vi "rsidr_core_global.vi"() -> ()   [LabVIEW 2020, in "Rohde&Schwarz CMWXP NR FR1 Measurement.lvlib"] (continued)
exceeding the specified power limits.\nDefault unit:  % \n\n<OffPowerBefore>\n float\nDefault unit:  dBm \n\n<OnPowerRMS>\n float\nDefault unit:  dBm \n\n<OnPowerPeak>\n float\nDefault unit:  dBm \n\n<OffPowerAfter>\n float\nDefault unit:  dBm\n\nAvailable Repeated Capabilities:\ninstance: i0, i1, i2, i3, i4, i5, i6, i7, i8, i9, i10, i11, i12, i13, i14, i15, i16, i17, i18, i19, i20, i21, i22, i23, i24, i25, i26, i27, i28, i29, i30, i31, i32\r\n\nRemote-control command(s):\nREAD:NRSub:MEAS<i>:MEValuation:PDYNamics:CURRent?"}, {"Level"=4, "Class Only"=FALSE, "Identifier"="RSCMWXPNRFR1M_ATTR_READ_MULTI_EVAL_MEAS_POWER_DYNAMICS_AVERAGE_RESULTS", "Descriptive Name"="Read Multi Eval Meas Power Dynamics Average Results", "Data Type"=enum."RawString", "Command"="READ:NRS:MEAS{instance}:MEV:PDYN:AVER?", "Access"=enum."Read Only", "Range Table"="", "Read Callback"="", "Write Callback"="", "Range Callback"="", "Check Callback"="", "Rngtable Callback"="", "Coerce Callback"="", "Supported Models"="", "Instrument Options"="", "Check Status Callback"="", "Flags"=0, "Help"="Return the average single value results of the power dynamics measurement.\n\nReturn values:  \n<Reliability>\n decimal\n\n<OutOfTolerance>\n decimal\nOut of tolerance result, i.e. percentage of measurement intervals of the statistic count for power dynamics measurements exceeding the specified power limits.\nDefault unit:  % \n\n<OffPowerBefore>\n float\nDefault unit:  dBm \n\n<OnPowerRMS>\n float\nDefault unit:  dBm \n\n<OnPowerPeak>\n float\nDefault unit:  dBm \n\n<OffPowerAfter>\n float\nDefault unit:  dBm\n\nAvailable Repeated Capabilities:\ninstance: i0, i1, i2, i3, i4, i5, i6, i7, i8, i9, i10, i11, i12, i13, i14, i15, i16, i17, i18, i19, i20, i21, i22, i23, i24, i25, i26, i27, i28, i29, i30, i31, i32\r\n\nRemote-control command(s):\nREAD:NRSub:MEAS<i>:MEValuation:PDYNamics:AVERage?"}, {"Level"=4, "Class Only"=FALSE, "Identifier"="RSCMWXPNRFR1M_ATTR_READ_MULTI_EVAL_MEAS_POWER_DYNAMICS_STANDARD_DEVIATION_RESULTS", "Descriptive Name"="Read Multi Eval Meas Power Dynamics Standard Deviation Results", "Data Type"=enum."RawString", "Command"="READ:NRS:MEAS{instance}:MEV:PDYN:SDEV?", "Access"=enum."Read Only", "Range Table"="", "Read Callback"="", "Write Callback"="", "Range Callback"="", "Check Callback"="", "Rngtable Callback"="", "Coerce Callback"="", "Supported Models"="", "Instrument Options"="", "Check Status Callback"="", "Flags"=0, "Help"="Return the standard deviation single value results of the power dynamics measurement.\n\nReturn values:  \n<Reliability>\n decimal\n\n<OutOfTolerance>\n decimal\nOut of tolerance result, i.e. percentage of measurement intervals of the statistic count for power dynamics measurements exceeding the specified power limits.\nDefault unit:  % \n\n<OffPowerBefore>\n float\nDefault unit:  dBm \n\n<OnPowerRMS>\n float\nDefault unit:  dBm \n\n<OnPowerPeak>\n float\nDefault unit:  dBm \n\n<OffPowerAfter>\n float\nDefault unit:  dBm\n\nAvailable Repeated Capabilities:\ninstance: i0, i1, i2, i3, i4, i5, i6, i7, i8, i9, i10, i11, i12, i13, i14, i15, i16, i17, i18, i19, i20, i21, i22, i23, i24, i25, i26, i27, i28, i29, i30, i31, i32\r\n\nRemote-control command(s):\nREAD:NRSub:MEAS<i>:MEValuation:PDYNamics:SDEViation?"}, {"Level"=4, "Class Only"=FALSE, "Identifier"="RSCMWXPNRFR1M_ATTR_READ_MULTI_EVAL_MEAS_POWER_DYNAMICS_MAXIMUM_RESULTS", "Descriptive Name"="Read Multi Eval Meas Power Dynamics Maximum Results", "Data Type"=enum."RawString", "Command"="READ:NRS:MEAS{instance}:MEV:PDYN:MAX?", "Access"=enum."Read Only", "Range Table"="", "Read Callback"="", "Write Callback"="", "Range Callback"="", "Check Callback"="", "Rngtable Callback"="", "Coerce Callback"="", "Supported Models"="", "Instrument Options"="", "Check Status Callback"="", "Flags"=0, "Help"="Return the maximum single value results of the power dynamics measurement.\n\nReturn values:  \n<Reliability>\n decimal\n\n<OutOfTolerance>\n decimal\nOut of tolerance result, i.e. percentage of measurement intervals of the statistic count for power dynamics measurements exceeding the specified power limits.\nDefault unit:  % \n\n<OffPowerBefore>\n float\nDefault unit:  dBm \n\n<OnPowerRMS>\n float\nDefault unit:  dBm \n\n<OnPowerPeak>\n float\nDefault unit:  dBm \n\n<OffPowerAfter>\n float\nDefault unit:  dBm\n\nAvailable Repeated Capabilities:\ninstance: i0, i1, i2, i3, i4, i5, i6, i7, i8, i9, i10, i11, i12, i13, i14, i15, i16, i17, i18, i19, i20, i21, i22, i23, i24, i25, i26, i27, i28, i29, i30, i31, i32\r\n\nRemote-control command(s):\nREAD:NRSub:MEAS<i>:MEValuation:PDYNamics:MAXimum?"}, {"Level"=4, "Class Only"=FALSE, "Identifier"="RSCMWXPNRFR1M_ATTR_READ_MULTI_EVAL_MEAS_POWER_DYNAMICS_MINIMUM_RESULTS", "Descriptive Name"="Read Multi Eval Meas Power Dynamics Minimum Results", "Data Type"=enum."RawString", "Command"="READ:NRS:MEAS{instance}:MEV:PDYN:MIN?", "Access"=enum."Read Only", "Range Table"="", "Read Callback"="", "Write Callback"="", "Range Callback"="", "Check Callback"="", "Rngtable Callback"="", "Coerce Callback"="", "Supported Models"="", "Instrument Options"="", "Check Status Callback"="", "Flags"=0, "Help"="Return the minimum single value results of the power dynamics measurement.\n\nReturn values:  \n<Reliability>\n decimal\n\n<OutOfTolerance>\n decimal\nOut of tolerance result, i.e. percentage of measurement intervals of the statistic count for power dynamics measurements exceeding the specified power limits.\nDefault unit:  % \n\n<OffPowerBefore>\n float\nDefault unit:  dBm \n\n<OnPowerRMS>\n float\nDefault unit:  dBm \n\n<OnPowerPeak>\n float\nDefault unit:  dBm \n\n<OffPowerAfter>\n float\nDefault unit:  dBm\n\nAvailable Repeated Capabilities:\ninstance: i0, i1, i2, i3, i4, i5, i6, i7, i8, i9, i10, i11, i12, i13, i14, i15, i16, i17, i18, i19, i20, i21, i22, i23, i24, i25, i26, i27, i28, i29, i30, i31, i32\r\n\nRemote-control command(s):\nREAD:NRSub:MEAS<i>:MEValuation:PDYNamics:MINimum?"}, {"Level"=4, "Class Only"=FALSE, "Identifier"="RSCMWXPNRFR1M_ATTR_FETCH_MULTI_EVAL_MEAS_POWER_DYNAMICS_CURRENT_RESULTS", "Descriptive Name"="Fetch Multi Eval Meas Power Dynamics Current Results", "Data Type"=enum."RawString", "Command"="FETC:NRS:MEAS{instance}:MEV:PDYN:CURR?", "Access"=enum."Read Only", "Range Table"="", "Read Callback"="", "Write Callback"="", "Range Callback"="", "Check Callback"="", "Rngtable Callback"="", "Coerce Callback"="", "Supported Models"="", "Instrument Options"="", "Check Status Callback"="", "Flags"=0, "Help"="Return the current single value results of the power dynamics measurement.\n\nReturn values:  \n<Reliability>\n decimal\n\n<OutOfTolerance>\n decimal\nOut of tolerance result, i.e. percentage of measurement intervals of the statistic count for power dynamics measurements exceeding the specified power limits.\nDefault unit:  % \n\n<OffPowerBefore>\n float\nDefault unit:  dBm \n\n<OnPowerRMS>\n float\nDefault unit:  dBm \n\n<OnPowerPeak>\n float\nDefault unit:  dBm \n\n<OffPowerAfter>\n float\nDefault unit:  dBm\n\nAvailable Repeated Capabilities:\ninstance: i0, i1, i2, i3, i4, i5, i6, i7, i8, i9, i10, i11, i12, i13, i14, i15, i16, i17, i18, i19, i20, i21, i22, i23, i24, i25, i26, i27, i28, i29, i30, i31, i32\r\n\nRemote-control command(s):\nFETCh:NRSub:MEAS<i>:MEValuation:PDYNamics:CURRent?"}, {"Level"=4, "Class Only"=FALSE, "Identifier"="RSCMWXPNRFR1M_ATTR_FETCH_MULTI_EVAL_MEAS_POWER_DYNAMICS_AVERAGE_RESULTS", "Descriptive Name"="Fetch Multi Eval Meas Power Dynamics Average Results", "Data Type"=enum."RawString", "Command"="FETC:NRS:MEAS{instance}:MEV:PDYN:AVER?", "Access"=enum."Read Only", "Range Table"="", "Read Callback"="", "Write Callback"="", "Range Callback"="", "Check Callback"="", "Rngtable Callback"="", "Coerce Callback"="", "Supported Models"="", "Instrument Options"="", "Check Status Callback"="", "Flags"=0, "Help"="Return the average single value results of the power dynamics measurement.\n\nReturn values:  \n<Reliability>\n decimal\n\n<OutOfTolerance>\n decimal\nOut of tolerance result, i.e. percentage of measurement intervals of the statistic count for power dynamics measurements exceeding the specified power limits.\nDefault unit:  % \n\n<OffPowerBefore>\n float\nDefault unit:  dBm \n\n<OnPowerRMS>\n float\nDefault unit:  dBm \n\n<OnPowerPeak>\n float\nDefault unit:  dBm \n\n<OffPowerAfter>\n float\nDefault unit:  dBm\n\nAvailable Repeated Capabilities:\ninstance: i0, i1, i2, i3, i4, i5, i6, i7, i8, i9, i10, i11, i12, i13, i14, i15, i16, i17, i18, i19, i20, i21, i22, i23, i24, i25, i26, i27, i28, i29, i30, i31, i32\r\n\nRemote-control command(s):\nFETCh:NRSub:MEAS<i>:MEValuation:PDYNamics:AVERage?"}, {"Level"=4, "Class Only"=FALSE, "Identifier"="RSCMWXPNRFR1M_ATTR_FETCH_MULTI_EVAL_MEAS_POWER_DYNAMICS_STANDARD_DEVIATION_RESULTS", "Descriptive Name"="Fetch Multi Eval Meas Power Dynamics Standard Deviation Results", "Data Type"=enum."RawString", "Command"="FETC:NRS:MEAS{instance}:MEV:PDYN:SDEV?", "Access"=enum."Read Only", "Range Table"="", "Read Callback"="", "Write Callback"="", "Range Callback"="", "Check Callback"="", "Rngtable Callback"="", "Coerce Callback"="", "Supported Models"="", "Instrument Options"="", "Check Status Callback"="", "Flags"=0, "Help"="Return the standard deviation single value results of the power dynamics measurement.\n\nReturn values:  \n<Reliability>\n decimal\n\n<OutOfTolerance>\n decimal\nOut of tolerance result, i.e. percentage of measurement intervals of the statistic count for power dynamics measurements exceeding the specified power limits.\nDefault unit:  % \n\n<OffPowerBefore>\n float\nDefault unit:  dBm \n\n<OnPowerRMS>\n float\nDefault unit:  dBm \n\n<OnPowerPeak>\n float\nDefault unit:  dBm \n\n<OffPowerAfter>\n float\nDefault unit:  dBm\n\nAvailable Repeated Capabilities:\ninstance: i0, i1, i2, i3, i4, i5, i6, i7, i8, i9, i10, i11, i12, i13, i14, i15, i16, i17, i18, i19, i20, i21, i22, i23, i24, i25, i26, i27, i28, i29, i30, i31, i32\r\n\nRemote-control command(s):\nFETCh:NRSub:MEAS<i>:MEValuation:PDYNamics:SDEViation?"}, {"Level"=4, "Class Only"=FALSE, "Identifier"="RSCMWXPNRFR1M_ATTR_FETCH_MULTI_EVAL_MEAS_POWER_DYNAMICS_MAXIMUM_RESULTS", "Descriptive Name"="Fetch Multi Eval Meas Power Dynamics Maximum Results", "Data Type"=enum."RawString", "Command"="FETC:NRS:MEAS{instance}:MEV:PDYN:MAX?", "Access"=enum."Read Only", "Range Table"="", "Read Callback"="", "Write Callback"="", "Range Callback"="", "Check Callback"="", "Rngtable Callback"="", "Coerce Callback"="", "Supported Models"="", "Instrument Options"="", "Check Status Callback"="", "Flags"=0, "Help"="Return the maximum single value results of the power dynamics measurement.\n\nReturn values:  \n<Reliability>\n decimal\n\n<OutOfTolerance>\n decimal\nOut of tolerance result, i.e. percentage of measurement intervals of the statistic count for power dynamics measurements exceeding the specified power limits.\nDefault unit:  % \n\n<OffPowerBefore>\n float\nDefault unit:  dBm \n\n<OnPowerRMS>\n float\nDefault unit:  dBm \n\n<OnPowerPeak>\n float\nDefault unit:  dBm \n\n<OffPowerAfter>\n float\nDefault unit:  dBm\n\nAvailable Repeated Capabilities:\ninstance: i0, i1, i2, i3, i4, i5, i6, i7, i8, i9, i10, i11, i12, i13, i14, i15, i16, i17, i18, i19, i20, i21, i22, i23, i24, i25, i26, i27, i28, i29, i30, i31, i32\r\n\nRemote-control command(s):\nFETCh:NRSub:MEAS<i>:MEValuation:PDYNamics:MAXimum?"}, {"Level"=4, "Class Only"=FALSE, "Identifier"="RSCMWXPNRFR1M_ATTR_FETCH_MULTI_EVAL_MEAS_POWER_DYNAMICS_MINIMUM_RESULTS", "Descriptive Name"="Fetch Multi Eval Meas Power Dynamics Minimum Results", "Data Type"=enum."RawString", "Command"="FETC:NRS:MEAS{instance}:MEV:PDYN:MIN?", "Access"=enum."Read Only", "Range Table"="", "Read Callback"="", "Write Callback"="", "Range Callback"="", "Check Callback"="", "Rngtable Callback"="", "Coerce Callback"="", "Supported Models"="", "Instrument Options"="", "Check Status Callback"="", "Flags"=0, "Help"="Return the minimum single value results of the power dynamics measurement.\n\nReturn values:  \n<Reliability>\n decimal\n\n<OutOfTolerance>\n decimal\nOut of tolerance result, i.e. percentage of measurement intervals of the statistic count for power dynamics measurements exceeding the specified power limits.\nDefault unit:  % \n\n<OffPowerBefore>\n float\nDefault unit:  dBm \n\n<OnPowerRMS>\n float\nDefault unit:  dBm \n\n<OnPowerPeak>\n float\nDefault unit:  dBm \n\n<OffPowerAfter>\n float\nDefault unit:  dBm\n\nAvailable Repeated Capabilities:\ninstance: i0, i1, i2, i3, i4, i5, i6, i7, i8, i9, i10, i11, i12, i13, i14, i15, i16, i17, i18, i19, i20, i21, i22, i23, i24, i25, i26, i27, i28, i29, i30, i31, i32\r\n\nRemote-control command(s):\nFETCh:NRSub:MEAS<i>:MEValuation:PDYNamics:MINimum?"}, {"Level"=3, "Class Only"=TRUE, "Identifier"="", "Descriptive Name"="List", "Data Type"=enum."ViInt32", "Command"="", "Access"=enum."Read Only", "Range Table"="", "Read Callback"="", "Write Callback"="", "Range Callback"="", "Check Callback"="", "Rngtable Callback"="", "Coerce Callback"="", "Supported Models"="", "Instrument Options"="", "Check Status Callback"="", "Flags"=0, "Help"="The attributes in this class return a selected list mode result for all measured segments. The number of returned results depends on the number of measured segments."}, {"Level"=4, "Class Only"=TRUE, "Identifier"="", "Descriptive Name"="ACLR Spectrum", "Data Type"=enum."ViInt32", "Command"="", "Access"=enum."Read Only", "Range Table"="", "Read Callback"="", "Write Callback"="", "Range Callback"="", "Check Callback"="", "Rngtable Callback"="", "Coerce Callback"="", "Supported Models"="", "Instrument Options"="", "Check Status Callback"="", "Flags"=0, "Help"="The attributes in this class return ACLR spectrum results for all measured segments. The number of returned results depends on the number of measured segments."}, {"Level"=5, "Class Only"=FALSE, "Identifier"="RSCMWXPNRFR1M_ATTR_FETCH_MULTI_EVAL_MEAS_LIST_ACLR_DETECTED_ALLOCATION_RESULTS", "Descriptive Name"="Fetch Multi Eval Meas List ACLR Detected Allocation Results", "Data Type"=enum."RawString", "Command"="FETC:NRS:MEAS{instance}:MEV:LIST:ACLR:DALL?", "Access"=enum."Read Only", "Range Table"="", "Read Callback"="", "Write Callback"="", "Range Callback"="", "Check Callback"="", "Rngtable Callback"="", "Coerce Callback"="", "Supported Models"="", "Instrument Options"="", "Check Status Callback"="", "Flags"=0, "Help"="Return the detected allocation for all measured list mode segments. The result is determined from the last measured slot of the statistical length of a segment. The individual measurements provide identical detected allocation results when measuring the same slot. However different statistical lengths can be defined for the measurements so that the measured slots and returned results can differ.\n\nThe results are returned as pairs per segment: <Reliability>, {<NrResBlocks>, <OffsetResBlocks>}seg 1, {<NrResBlocks>, <OffsetResBlocks>}seg 2, ...\n\nReturn values:  \n<Reliability>\n decimal\n\n<NrResBlocks>\n decimal\nNumber of allocated resource blocks\n\n<OffsetResBlocks>\n decimal\nOffset of the first allocated resource block from the edge of the allocated UL transmission bandwidth\n\nAvailable Repeated Capabilities:\ninstance: i0, i1, i2, i3, i4, i5, i6, i7, i8, i9, i10, i11, i12, i13, i14, i15, i16, i17, i18, i19, i20, i21, i22, i23, i24, i25, i26, i27, i28, i29, i30, i31, i32\r\n\nRemote-control command(s):\nFETCh:NRSub:MEAS<i>:MEValuation:LIST:ACLR:DALLocation?"}, {"Level"=5, "Class Only"=FALSE, "Identifier"="RSCMWXPNRFR1M_ATTR_FETCH_MULTI_EVAL_MEAS_LIST_ACLR_NR_CURRENT_RESULTS", "Descriptive Name"="Fetch Multi Eval Meas List ACLR NR Current Results", "Data Type"=enum."RawString", "Command"="FETC:NRS:MEAS{instance}:MEV:LIST:ACLR:NR:CURR?", "Access"=enum."Read Only", "Range Table"="", "Read Callback"="", "Write Callback"="", "Range Callback"="", "Check Callback"="", "Rngtable Callback"="", "Coerce Callback"="", "Supported Models"="", "Instrument Options"="", "Check Status Callback"="", "Flags"=0, "Help"="Return the power in the allocated NR channel for all measured list mode segments.\n\nReturn values:  \n<Reliability>\n decimal\n\n<Power>\n float\nComma-separated list of values, one per measured segment\nDefault unit:  dBm\n\nAvailable Repeated Capabilities:\ninstance: i0, i1, i2, i3, i4, i5, i6, i7, i8, i9, i10, i11, i12, i13, i14, i15, i16, i17, i18, i19, i20, i21, i22, i23, i24, i25, i26, i27, i28, i29, i30, i31, i32\r\n\nRemote-control command(s):\nFETCh:NRSub:MEAS<i>:MEValuation:LIST:ACLR:NR:CURRent?"}, {"Level"=5, "Class Only"=FALSE, "Identifier"="RSCMWXPNRFR1M_ATTR_FETCH_MULTI_EVAL_MEAS_LIST_ACLR_NR_AVERAGE_RESULTS", "Descriptive Name"="Fetch Multi Eval Meas List ACLR NR Average Results", "Data Type"=enum."RawString", "Command"="FETC:NRS:MEAS{instance}:MEV:LIST:ACLR:NR:AVER?", "Access"=enum."Read Only", "Range Table"="", "Read Callback"="", "Write Callback"="", "Range Callback"="", "Check Callback"="", "Rngtable Callback"="", "Coerce Callback"="", "Supported Models"="", "Instrument Options"="", "Check Status Callback"="", "Flags"=0, "Help"="Return the average power in the allocated NR channel for all measured list mode segments.\n\nReturn values:  \n<Reliability>\n decimal\n\n<Power>\n float\nComma-separated list of values, one per measured segment\nDefault unit:  dBm\n\nAvailable Repeated Capabilities:\ninstance: i0, i1, i2, i3, i4, i5, i6, i7, i8, i9, i10, i11, i12, i13, i14, i15, i16, i17, i18, i19, i20, i21, i22, i23, i24, i25, i26, i27, i28, i29, i30, i31, i32\r\n\nRemote-control command(s):\nFETCh:NRSub:MEAS<i>:MEValuation:LIST:ACLR:NR:AVERage?"}, {"Level"=5, "Class Only"=FALSE, "Identifier"="RSCMWXPNRFR1M_ATTR_QUERY_MULTI_EVAL_MEAS_LIST_ACLR_NR_CURRENT_LIMIT_CHECK_RESULTS", "Descriptive Name"="Query Multi Eval Meas List ACLR NR Current Limit Check Results", "Data Type"=enum."RawString", "Command"="CALC:NRS:MEAS{instance}:MEV:LIST:ACLR:NR:CURR?", "Access"=enum."Read Only", "Range Table"="", "Read Callback"="", "Write Callback"="", "Range Callback"="", "Check Callback"="", "Rngtable Callback"="", "Coerce Callback"="", "Supported Models"="", "Instrument Options"="", "Check Status Callback"="", "Flags"=0, "Help"="Return the power limit check results in the allocated NR channel for all measured list mode segments.\n\nReturn values:  \n<Reliability>\n decimal\n\n<PowerLimCheck>\n limit check result\nComma-separated list of results, one per measured segment\n\nAvailable Repeated Capabilities:\ninstance: i0, i1, i2, i3, i4, i5, i6, i7, i8, i9, i10, i11, i12, i13, i14, i15, i16, i17, i18, i19, i20, i21, i22, i23, i24, i25, i26, i27, i28, i29, i30, i31, i32\r\n\nRemote-control command(s):\nCALCulate:NRSub:MEAS<i>:MEValuation:LIST:ACLR:NR:CURRent?"}, {"Level"=5, "Class Only"=FALSE, "Identifier"="RSCMWXPNRFR1M_ATTR_QUERY_MULTI_EVAL_MEAS_LIST_ACLR_NR_AVERAGE_LIMIT_CHECK_RESULTS", "Descriptive Name"="Query Multi Eval Meas List ACLR NR Average Limit Check Results", "Data Type"=enum."RawString", "Command"="CALC:NRS:MEAS{instance}:MEV:LIST:ACLR:NR:AVER?", "Access"=enum."Read Only", "Range Table"="", "Read Callback"="", "Write Callback"="", "Range Callback"="", "Check Callback"="", "Rngtable Callback"="", "Coerce Callback"="", "Supported Models"="", "Instrument Options"="", "Check Status Callback"="", "Flags"=0, "Help"="Return the average \tpower limit check results in the allocated NR channel for all measured list mode segments.\n\nReturn values:  \n<Reliability>\n decimal\n\n<PowerLimCheck>\n limit check result\nComma-separated list of results, one per measured segment\n\nAvailable Repeated Capabilities:\ninstance: i0, i1, i2, i3, i4, i5, i6, i7, i8, i9, i10, i11, i12, i13, i14, i15, i16, i17, i18, i19, i20, i21, i22, i23, i24, i25, i26, i27, i28, i29, i30, i31, i32\r\n\nRemote-control command(s):\nCALCulate:NRSub:MEAS<i>:MEValuation:LIST:ACLR:NR:AVERage?"}, {"Level"=5, "Class Only"=FALSE, "Identifier"="RSCMWXPNRFR1M_ATTR_FETCH_MULTI_EVAL_MEAS_LIST_ACLR_NR_NEGATIVE_CURRENT_RESULTS", "Descriptive Name"="Fetch Multi Eval Meas List ACLR NR Negative Current Results", "Data Type"=enum."RawString", "Command"="FETC:NRS:MEAS{instance}:MEV:LIST:ACLR:NR:NEG:CURR?", "Access"=enum."Read Only", "Range Table"="", "Read Callback"="", "Write Callback"="", "Range Callback"="", "Check Callback"="", "Rngtable Callback"="", "Coerce Callback"="", "Supported Models"="", "Instrument Options"="", "Check Status Callback"="", "Flags"=0, "Help"="Return the ACLR for the first adjacent NR channel below (Negative) the carrier frequency for all measured list mode segments.\n\nReturn values:  \n<Reliability>\n decimal\n\n<ACLR>\n float\nComma-separated list of values, one per measured segment\nDefault unit:  dB\n\nAvailable Repeated Capabilities:\ninstance: i0, i1, i2, i3, i4, i5, i6, i7, i8, i9, i10, i11, i12, i13, i14, i15, i16, i17, i18, i19, i20, i21, i22, i23, i24, i25, i26, i27, i28, i29, i30, i31, i32\r\n\nRemote-control command(s):\nFETCh:NRSub:MEAS<i>:MEValuation:LIST:ACLR:NR:NEGativ:CURRent?"}, {"Level"=5, "Class Only"=FALSE, "Identifier"="RSCMWXPNRFR1M_ATTR_FETCH_MULTI_EVAL_MEAS_LIST_ACLR_NR_NEGATIVE_AVERAGE_RESULTS", "Descriptive Name"="Fetch Multi Eval Meas List ACLR NR Negative Average Results", "Data Type"=enum."RawString", "Command"="FETC:NRS:MEAS{instance}:MEV:LIST:ACLR:NR:NEG:AVER?", "Access"=enum."Read Only", "Range Table"="", "Read Callback"="", "Write Callback"="", "Range Callback"="", "Check Callback"="", "Rngtable Callback"="", "Coerce Callback"="", "Supported Models"="", "Instrument Options"="", "Check Status Callback"="", "Flags"=0, "Help"="Return the average ACLR for the first adjacent NR channel below (Negative) the carrier frequency for all measured list mode segments.\n\nReturn values:  \n<Reliability>\n decimal\n\n<ACLR>\n float\nComma-separated list of values, one per measured segment\nDefault unit:  dB\n\nAvailable Repeated Capabilities:\ninstance: i0, i1, i2, i3, i4, i5, i6, i7, i8, i9, i10, i11, i12, i13, i14, i15, i16, i17, i18, i19, i20, i21, i22, i23, i24, i25, i26, i27, i28, i29, i30, i31, i32\r\n\nRemote-control command(s):\nFETCh:NRSub:MEAS<i>:MEValuation:LIST:ACLR:NR:NEGativ:AVERage?"}, {"Level"=5, "Class Only"=FALSE, "Identifier"="RSCMWXPNRFR1M_ATTR_FETCH_MULTI_EVAL_MEAS_LIST_ACLR_NR_POSITIVE_CURRENT_RESULTS", "Descriptive Name"="Fetch Multi Eval Meas List ACLR NR Positive Current Results", "Data Type"=enum."RawString", "Command"="FETC:NRS:MEAS{instance}:MEV:LIST:ACLR:NR:POS:CURR?", "Access"=enum."Read Only", "Range Table"="", "Read Callback"="", "Write Callback"="", "Range Callback"="", "Check Callback"="", "Rngtable Callback"="", "Coerce Callback"="", "Supported Models"="", "Instrument Options"="", "Check Status Callback"="", "Flags"=0, "Help"="Return the ACLR for the first adjacent NR channel above (Positive) the carrier frequency for all measured list mode segments.\n\nReturn values:  \n<Reliability>\n decimal\n\n<ACLR>\n float\nComma-separated list of values, one per measured segment\nDefault unit:  dB\n\nAvailable Repeated Capabilities:\ninstance: i0, i1, i2, i3, i4, i5, i6, i7, i8, i9, i10, i11, i12, i13, i14, i15, i16, i17, i18, i19, i20, i21, i22, i23, i24, i25, i26, i27, i28, i29, i30, i31, i32\r\n\nRemote-control command(s):\nFETCh:NRSub:MEAS<i>:MEValuation:LIST:ACLR:NR:POSitiv:CURRent?"}, {"Level"=5, "Class Only"=FALSE, "Identifier"="RSCMWXPNRFR1M_ATTR_FETCH_MULTI_EVAL_MEAS_LIST_ACLR_NR_POSITIVE_AVERAGE_RESULTS", "Descriptive Name"="Fetch Multi Eval Meas List ACLR NR Positive Average Results", "Data Type"=enum."RawString", "Command"="FETC:NRS:MEAS{instance}:MEV:LIST:ACLR:NR:POS:AVER?", "Access"=enum."Read Only", "Range Table"="", "Read Callback"="", "Write Callback"="", "Range Callback"="", "Check Callback"="", "Rngtable Callback"="", "Coerce Callback"="", "Supported Models"="", "Instrument Options"="", "Check Status Callback"="", "Flags"=0, "Help"="Return the average ACLR for the first adjacent NR channel above (Positive) the carrier frequency for all measured list mode segments.\n\nReturn values:  \n<Reliability>\n decimal\n\n<ACLR>\n float\nComma-separated list of values, one per measured segment\nDefault unit:  dB\n\nAvailable Repeated Capabilities:\ninstance: i0, i1, i2, i3, i4, i5, i6, i7, i8, i9, i10, i11, i12, i13, i14, i15, i16, i17, i18, i19, i20, i21, i22, i23, i24, i25, i26, i27, i28, i29, i30, i31, i32\r\n\nRemote-control command(s):\nFETCh:NRSub:MEAS<i>:MEValuation:LIST:ACLR:NR:POSitiv:AVERage?"}, {"Level"=5, "Class Only"=FALSE, "Identifier"="RSCMWXPNRFR1M_ATTR_QUERY_MULTI_EVAL_MEAS_LIST_ACLR_NR_NEGATIVE_CURRENT_LIMIT_CHECK_RESULTS", "Descriptive Name"="Query Multi Eval Meas List ACLR NR Negative Current Limit Check Results", "Data Type"=enum."RawString", "Command"="CALC:NRS:MEAS{instance}:MEV:LIST:ACLR:NR:NEG:CURR?", "Access"=enum."Read Only", "Range Table"="", "Read Callback"="", "Write Callback"="", "Range Callback"="", "Check Callback"="", "Rngtable Callback"="", "Coerce Callback"="", "Supported Models"="", "Instrument Options"="", "Check Status Callback"="", "Flags"=0, "Help"="Return the ACLR limit check results for the first adjacent NR channel below (Negative) the carrier frequency for all measured list mode segments.\n\nReturn values:  \n<Reliability>\n decimal\n\n<ACLRLimCheck>\n limit check result\nComma-separated list of values, one per measured segment\n\nAvailable Repeated Capabilities:\ninstance: i0, i1, i2, i3, i4, i5, i6, i7, i8, i9, i10, i11, i12, i13, i14, i15, i16, i17, i18, i19, i20, i21, i22, i23, i24, i25, i26, i27, i28, i29, i30, i31, i32\r\n\nRemote-control command(s):\nCALCulate:NRSub:MEAS<i>:MEValuation:LIST:ACLR:NR:NEGativ:CURRent?"}, {"Level"=5, "Class Only"=FALSE, "Identifier"="RSCMWXPNRFR1M_ATTR_QUERY_MULTI_EVAL_MEAS_LIST_ACLR_NR_NEGATIVE_AVERAGE_LIMIT_CHECK_RESULTS", "Descriptive Name"="Query Multi Eval Meas List ACLR NR Negative Average Limit Check Results", "Data Type"=enum."RawString", "Command"="CALC:NRS:MEAS{instance}:MEV:LIST:ACLR:NR:NEG:AVER?", "Access"=enum."Read Only", "Range Table"="", "Read Callback"="", "Write Callback"="", "Range Callback"="", "Check Callback"="", "Rngtable Callback"="", "Coerce Callback"="", "Supported Models"="", "Instrument Options"="", "Check Status Callback"="", "Flags"=0, "Help"="Return the average ACLR limit check results for the first adjacent NR channel below (Negative) the carrier frequency for all measured list mode segments.\n\nReturn values:  \n<Reliability>\n decimal\n\n<ACLRLimCheck>\n limit check result\nComma-separated list of values, one per measured segment\n\nAvailable Repeated Capabilities:\ninstance: i0, i1, i2, i3, i4, i5, i6, i7, i8, i9, i10, i11, i12, i13, i14, i15, i16, i17, i18, i19, i20, i21, i22, i23, i24, i25, i26, i27, i28, i29, i30, i31, i32\r\n\nRemote-control command(s):\nCALCulate:NRSub:MEAS<i>:MEValuation:LIST:ACLR:NR:NEGativ:AVERage?"}, {"Level"=5, "Class Only"=FALSE, "Identifier"="RSCMWXPNRFR1M_ATTR_QUERY_MULTI_EVAL_MEAS_LIST_ACLR_NR_POSITIVE_CURRENT_LIMIT_CHECK_RESULTS", "Descriptive Name"="Query Multi Eval Meas List ACLR NR Positive Current Limit Check Results", "Data Type"=enum."RawString", "Command"="CALC:NRS:MEAS{instance}:MEV:LIST:ACLR:NR:POS:CURR?", "Access"=enum."Read Only", "Range Table"="", "Read Callback"="", "Write Callback"="", "Range Callback"="", "Check Callback"="", "Rngtable Callback"="", "Coerce Callback"="", "Supported Models"="", "Instrument Options"="", "Check Status Callback"="", "Flags"=0, "Help"="Return the ACLR limit check results for the first adjacent NR channel above (Positive) the carrier frequency for all measured list mode segments.\n\nReturn values:  \n<Reliability>\n decimal\n\n<ACLRLimCheck>\n limit check result\nComma-separated list of values, one per measured segment\n\nAvailable Repeated Capabilities:\ninstance: i0, i1, i2, i3, i4, i5, i6, i7, i8, i9, i10, i11, i12, i13, i14, i15, i16, i17, i18, i19, i20, i21, i22, i23, i24, i25, i26, i27, i28, i29, i30, i31, i32\r\n\nRemote-control command(s):\nCALCulate:NRSub:MEAS<i>:MEValuation:LIST:ACLR:NR:POSitiv:CURRent?"}, {"Level"=5, "Class Only"=FALSE, "Identifier"="RSCMWXPNRFR1M_ATTR_QUERY_MULTI_EVAL_MEAS_LIST_ACLR_NR_POSITIVE_AVERAGE_LIMIT_CHECK_RESULTS", "Descriptive Name"="Query Multi Eval Meas List ACLR NR Positive Average Limit Check Results", "Data Type"=enum."RawString", "Command"="CALC:NRS:MEAS{instance}:MEV:LIST:ACLR:NR:POS:AVER?", "Access"=enum."Read Only", "Range Table"="", "Read Callback"="", "Write Callback"="", "Range Callback"="", "Check Callback"="", "Rngtable Callback"="", "Coerce Callback"="", "Supported Models"="", "Instrument Options"="", "Check Status Callback"="", "Flags"=0, "Help"="Return the average ACLR limit check results for the first adjacent NR channel above (Positive) the carrier frequency for all measured list mode segments.\n\nReturn values:  \n<Reliability>\n decimal\n\n<ACLRLimCheck>\n limit check result\nComma-separated list of values, one per measured segment\n\nAvailable Repeated Capabilities:\ninstance: i0, i1, i2, i3, i4, i5, i6, i7, i8, i9, i10, i11, i12, i13, i14, i15, i16, i17, i18, i19, i20, i21, i22, i23, i24, i25, i26, i27, i28, i29, i30, i31, i32\r\n\nRemote-control command(s):\nCALCulate:NRSub:MEAS<i>:MEValuation:LIST:ACLR:NR:POSitiv:AVERage?"}, {"Level"=5, "Class Only"=TRUE, "Identifier"="", "Descriptive Name"="UTRA", "Data Type"=enum."ViInt32", "Command"="", "Access"=enum."Read Only", "Range Table"="", "Read Callback"="", "Write Callback"="", "Range Callback"="", "Check Callback"="", "Rngtable Callback"="", "Coerce Callback"="", "Supported Models"="", "Instrument Options"="", "Check Status Callback"="", "Flags"=0, "Help"="The attributes in this class return results for adjacent UTRA channels."}, {"Level"=6, "Class Only"=FALSE, "Identifier"="RSCMWXPNRFR1M_ATTR_FETCH_MULTI_EVAL_MEAS_LIST_ACLR_UTRA_NEGATIVE_CURRENT_RESULTS", "Descriptive Name"="Fetch Multi Eval Meas List ACLR UTRA Negative Current Results", "Data Type"=enum."RawString", "Command"="FETC:NRS:MEAS{instance}:MEV:LIST:ACLR:UTRA{UTRA}:NEG:CURR?", "Access"=enum."Read Only", "Range Table"="", "Read Callback"="", "Write Callback"="", "Range Callback"="", "Check Callback"="", "Rngtable Callback"="", "Coerce Callback"="", "Supported Models"="", "Instrument Options"="", "Check Status Callback"="", "Flags"=0, "Help"="Return the ACLR for the first or second adjacent UTRA channel below (Negative) the carrier frequency for all measured list mode segments.\n\nReturn values:  \n<Reliability>\n decimal\n\n<ACLR>\n float\nComma-separated list of values, one per measured segment\nDefault unit:  dB\n\nAvailable Repeated Capabilities:\ninstance: i0, i1, i2, i3, i4, i5, i6, i7, i8, i9, i10, i11, i12, i13, i14, i15, i16, i17, i18, i19, i20, i21, i22, i23, i24, i25, i26, i27, i28, i29, i30, i31, i32\r\nUTRA: UTRA1, UTRA2\r\n\nRemote-control command(s):\nFETCh:NRSub:MEAS<i>:MEValuation:LIST:ACLR:UTRA<no>:NEGativ:CURRent?"}, {"Level"=6, "Class Only"=FALSE, "Identifier"="RSCMWXPNRFR1M_ATTR_FETCH_MULTI_EVAL_MEAS_LIST_ACLR_UTRA_NEGATIVE_AVERAGE_RESULTS", "Descriptive Name"="Fetch Multi Eval Meas List ACLR UTRA Negative Average Results", "Data Type"=enum."RawString", "Command"="FETC:NRS:MEAS{instance}:MEV:LIST:ACLR:UTRA{UTRA}:NEG:AVER?", "Access"=enum."Read Only", "Range Table"="", "Read Callback"="", "Write Callback"="", "Range Callback"="", "Check Callback"="", "Rngtable Callback"="", "Coerce Callback"="", "Supported Models"="", "Instrument Options"="", "Check Status Callback"="", "Flags"=0, "Help"="Return the average ACLR for the first or second adjacent UTRA channel below (Negative) the carrier frequency for all measured list mode segments.\n\nReturn values:  \n<Reliability>\n decimal\n\n<ACLR>\n float\nComma-separated list of values, one per measured segment\nDefault unit:  dB\n\nAvailable Repeated Capabilities:\ninstance: i0, i1, i2, i3, i4, i5, i6, i7, i8, i9, i10, i11, i12, i13, i14, i15, i16, i17, i18, i19, i20, i21, i22, i23, i24, i25, i26, i27, i28, i29, i30, i31, i32\r\nUTRA: UTRA1, UTRA2\r\n\nRemote-control command(s):\nFETCh:NRSub:MEAS<i>:MEValuation:LIST:ACLR:UTRA<no>:NEGativ:AVERage?"}, {"Level"=6, "Class Only"=FALSE, "Identifier"="RSCMWXPNRFR1M_ATTR_FETCH_MULTI_EVAL_MEAS_LIST_ACLR_UTRA_POSITIVE_CURRENT_RESULTS", "Descriptive Name"="Fetch Multi Eval Meas List ACLR UTRA Positive Current Results", "Data Type"=enum."RawString", "Command"="FETC:NRS:MEAS{instance}:MEV:LIST:ACLR:UTRA{UTRA}:POS:CURR?", "Access"=enum."Read Only", "Range Table"="", "Read Callback"="", "Write Callback"="", "Range Callback"="", "Check Callback"="", "Rngtable Callback"="", "Coerce Callback"="", "Supported Models"="", "Instrument Options"="", "Check Status Callback"="", "Flags"=0, "Help"="Return the ACLR for the first or second adjacent UTRA channel above (Positive) the carrier frequency for all measured list mode segments.\n\nReturn values:  \n<Reliability>\n decimal\n\n<ACLR>\n float\nComma-separated list of values, one per measured segment\nDefault unit:  dB\n\nAvailable Repeated Capabilities:\ninstance: i0, i1, i2, i3, i4, i5, i6, i7, i8, i9, i10, i11, i12, i13, i14, i15, i16, i17, i18, i19, i20, i21, i22, i23, i24, i25, i26, i27, i28, i29, i30, i31, i32\r\nUTRA: UTRA1, UTRA2\r\n\nRemote-control command(s):\nFETCh:NRSub:MEAS<i>:MEValuation:LIST:ACLR:UTRA<no>:POSitiv:CURRent?"}, {"Level"=6, "Class Only"=FALSE, "Identifier"="RSCMWXPNRFR1M_ATTR_FETCH_MULTI_EVAL_MEAS_LIST_ACLR_UTRA_POSITIVE_AVERAGE_RESULTS", "Descriptive Name"="Fetch Multi Eval Meas List ACLR UTRA Positive Average Results", "Data Type"=enum."RawString", "Command"="FETC:NRS:MEAS{instance}:MEV:LIST:ACLR:UTRA{UTRA}:POS:AVER?", "Access"=enum."Read Only", "Range Table"="", "Read Callback"="", "Write Callback"="", "Range Callback"="", "Check Callback"="", "Rngtable Callback"="", "Coerce Callback"="", "Supported Models"="", "Instrument Options"="", "Check Status Callback"="", "Flags"=0, "Help"="Return the average ACLR for the first or second adjacent UTRA channel above (Positive) the carrier frequency for all measured list mode segments.\n\nReturn values:  \n<Reliability>\n decimal\n\n<ACLR>\n float\nComma-separated list of values, one per measured segment\nDefault unit:  dB\n\nAvailable Repeated Capabilities:\ninstance: i0, i1, i2, i3, i4, i5, i6, i7, i8, i9, i10, i11, i12, i13, i14, i15, i16, i17, i18, i19, i20, i21, i22, i23, i24, i25, i26, i27, i28, i29, i30, i31, i32\r\nUTRA: UTRA1, UTRA2\r\n\nRemote-control command(s):\nFETCh:NRSub:MEAS<i>:MEValuation:LIST:ACLR:UTRA<no>:POSitiv:AVERage?"}, {"Level"=6, "Class Only"=FALSE, "Identifier"="RSCMWXPNRFR1M_ATTR_QUERY_MULTI_EVAL_MEAS_LIST_ACLR_UTRA_NEGATIVE_CURRENT_LIMIT_CHECK_RESULTS", "Descriptive Name"="Query Multi Eval Meas List ACLR UTRA Negative Current Limit Check Results", "Data Type"=enum."RawString", "Command"="CALC:NRS:MEAS{instance}:MEV:LIST:ACLR:UTRA{UTRA}:NEG:CURR?", "Access"=enum."Read Only", "Range Table"="", "Read Callback"="", "Write Callback"="", "Range Callback"="", "Check Callback"="", "Rngtable Callback"="", "Coerce Callback"="", "Supported Models"="", "Instrument Options"="", "Check Status Callback"="", "Flags"=0, "Help"="Return the ACLR limit check results for the first or second adjacent UTRA channel below (Negative) the carrier frequency for all measured list mode segments.\n\nReturn values:  \n<Reliability>\n decimal\n\n<ACLRLimCheck>\n limit check result\nComma-separated list of values, one per measured segment\n\nAvailable Repeated Capabilities:\ninstance: i0, i1, i2, i3, i4, i5, i6, i7, i8, i9, i10, i11, i12, i13, i14, i15, i16, i17, i18, i19, i20, i21, i22, i23, i24, i25, i26, i27, i28, i29, i30, i31, i32\r\nUTRA: UTRA1, UTRA2\r\n\nRemote-control command(s):\nCALCulate:NRSub:MEAS<i>:MEValuation:LIST:ACLR:UTRA<no>:NEGativ:CURRent?"}, {"Level"=6, "Class Only"=FALSE, "Identifier"="RSCMWXPNRFR1M_ATTR_QUERY_MULTI_EVAL_MEAS_LIST_ACLR_UTRA_NEGATIVE_AVERAGE_LIMIT_CHECK_RESULTS", "Descriptive Name"="Query Multi Eval Meas List ACLR UTRA Negative Average Limit Check Results", "Data Type"=enum."RawString", "Command"="CALC:NRS:MEAS{instance}:MEV:LIST:ACLR:UTRA{UTRA}:NEG:AVER?", "Access"=enum."Read Only", "Range Table"="", "Read Callback"="", "Write Callback"="", "Range Callback"="", "Check Callback"="", "Rngtable Callback"="", "Coerce Callback"="", "Supported Models"="", "Instrument Options"="", "Check Status Callback"="", "Flags"=0, "Help"="Return the average ACLR limit check results for the first or second adjacent UTRA channel below (Negative) the carrier frequency for all measured list mode segments.\n\nReturn values:  \n<Reliability>\n decimal\n\n<ACLRLimCheck>\n limit check result\nComma-separated list of values, one per measured segment\n\nAvailable Repeated Capabilities:\ninstance: i0, i1, i2, i3, i4, i5, i6, i7, i8, i9, i10, i11, i12, i13, i14, i15, i16, i17, i18, i19, i20, i21, i22, i23, i24, i25, i26, i27, i28, i29, i30, i31, i32\r\nUTRA: UTRA1, UTRA2\r\n\nRemote-control command(s):\nCALCulate:NRSub:MEAS<i>:MEValuation:LIST:ACLR:UTRA<no>:NEGativ:AVERage?"}, {"Level"=6, "Class Only"=FALSE, "Identifier"="RSCMWXPNRFR1M_ATTR_QUERY_MULTI_EVAL_MEAS_LIST_ACLR_UTRA_POSITIVE_CURRENT_LIMIT_CHECK_RESULTS", "Descriptive Name"="Query Multi Eval Meas List ACLR UTRA Positive Current Limit Check Results", "Data Type"=enum."RawString", "Command"="CALC:NRS:MEAS{instance}:MEV:LIST:ACLR:UTRA{UTRA}:POS:CURR?", "Access"=enum."Read Only", "Range Table"="", "Read Callback"="", "Write Callback"="", "Range Callback"="", "Check Callback"="", "Rngtable Callback"="", "Coerce Callback"="", "Supported Models"="", "Instrument Options"="", "Check Status Callback"="", "Flags"=0, "Help"="Return the ACLR limit check results for the first or second adjacent UTRA channel above (Positive) the carrier frequency for all measured list mode segments.\n\nReturn values:  \n<Reliability>\n decimal\n\n<ACLRLimCheck>\n limit check result\nComma-separated list of values, one per measured segment\n\nAvailable Repeated Capabilities:\ninstance: i0, i1, i2, i3, i4, i5, i6, i7, i8, i9, i10, i11, i12, i13, i14, i15, i16, i17, i18, i19, i20, i21, i22, i23, i24, i25, i26, i27, i28, i29, i30, i31, i32\r\nUTRA: UTRA1, UTRA2\r\n\nRemote-control command(s):\nCALCulate:NRSub:MEAS<i>:MEValuation:LIST:ACLR:UTRA<no>:POSitiv:CURRent?"}, {"Level"=6, "Class Only"=FALSE, "Identifier"="RSCMWXPNRFR1M_ATTR_QUERY_MULTI_EVAL_MEAS_LIST_ACLR_UTRA_POSITIVE_AVERAGE_LIMIT_CHECK_RESULTS", "Descriptive Name"="Query Multi Eval Meas List ACLR UTRA Positive Average Limit Check Results", "Data Type"=enum."RawString", "Command"="CALC:NRS:MEAS{instance}:MEV:LIST:ACLR:UTRA{UTRA}:POS:AVER?", "Access"=enum."Read Only", "Range Table"="", "Read Callback"="", "Write Callback"="", "Range Callback"="", "Check Callback"="", "Rngtable Callback"="", "Coerce Callback"="", "Supported Models"="", "Instrument Options"="", "Check Status Callback"="", "Flags"=0, "Help"="Return the average ACLR limit check results for the first or second adjacent UTRA channel above (Positive) the carrier frequency for all measured list mode segments.\n\nReturn values:  \n<Reliability>\n decimal\n\n<ACLRLimCheck>\n limit check result\nComma-separated list of values, one per measured segment\n\nAvailable Repeated Capabilities:\ninstance: i0, i1, i2, i3, i4, i5, i6, i7, i8, i9, i10, i11, i12, i13, i14, i15, i16, i17, i18, i19, i20, i21, i22, i23, i24, i25, i26, i27, i28, i29, i30, i31, i32\r\nUTRA: UTRA1, UTRA2\r\n\nRemote-control command(s):\nCALCulate:NRSub:MEAS<i>:MEValuation:LIST:ACLR:UTRA<no>:POSitiv:AVERage?"}, {"Level"=4, "Class Only"=TRUE, "Identifier"="", "Descriptive Name"="Equalizer Spectrum Flatness", "Data Type"=enum."ViInt32", "Command"="", "Access"=enum."Read Only", "Range Table"="", "Read Callback"="", "Write Callback"="", "Range Callback"="", "Check Callback"="", "Rngtable Callback"="", "Coerce Callback"="", "Supported Models"="", "Instrument Options"="", "Check Status Callback"="", "Flags"=0, "Help"="The attributes in this class return equalizer spectrum flatness results for all measured segments. The number of returned results depends on the number of measured segments."}, 
